vi "listenUDP.vi"(8 "error in (no error)":errorcluster, 11 "UDP Network Connection in":refnum<k16>) -> (0 "error out":errorcluster, 2 "data out":string, 3 "UDP Network Connection out":refnum<k16>)   [LabVIEW 2017, in "communicateMLC.lvlib"]
doc: "This VI listens for UDP data from the PC. The listening port is 60006."
uses:
  communicateMLC.lvlib
  TypeDefs/UDPListenFGV.ctl
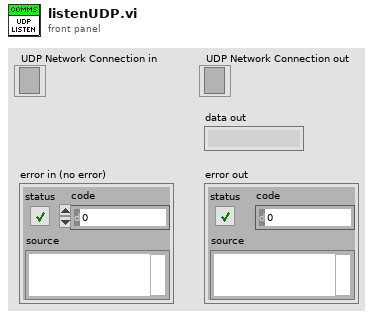
[diagram p1: front panel]
types:
  T1 = typedef "communicateMLC.lvlib/UDPListenFGV.ctl" = enum16{"Write", "Read"}
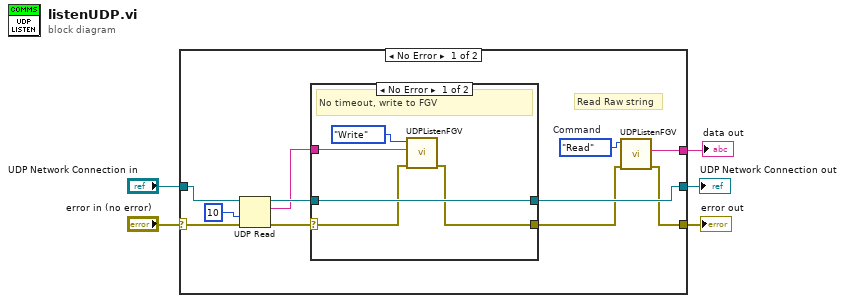
[diagram p0: block diagram]
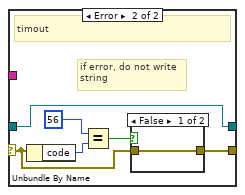
[diagram p2: hidden frame]
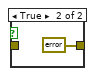
[diagram p3: hidden frame]
diagram:
  n1 = case shown="No Error" "error in (no error)" {
    selector: "error in (no error)" -> [w11 w31]
    tunnel: [w16 w30] -> w5
    tunnel: [w6 w31] -> w4
    tunnel: "UDP Network Connection in" -> [w15 w30]
    tunnel: [w8 _] -> w1
    frame No Error {
      w9 = UDPListenFGV."Read"  # Command
      # "Read Raw string"
      n2 = UDP Read(connection ID=w15, timeout ms (25000)=10, 8:w11) -> (data out=w10:string, error out=w13:errorcluster, 3:w14:refnum<k16>)  [unwired: 1 in, 2 out]
      n3 = case shown="No Error" w13 {
        selector: w13 -> [w20 w23]
        tunnel: w14 -> [w21 w22]
        tunnel: w10 -> [w18 _]
        tunnel: [w19 w24] -> w7
        tunnel: [w21 w22] -> w16
        frame No Error {
          # "No timeout, write to FGV"
          n4 = call "UDPListenFGV.vi"("error in (no error)"=w20, "Write Data"=w18, "Command"=UDPListenFGV."Write") -> ("error out"=w19:errorcluster)  [unwired: 7 in, 1 out]
        }
        frame Error {
          # "if error, do not write\nstring"
          # "timout"
          n5 = Unbundle By Name(w23) -> ("code"=w27:i32)
          n6 = Equal?(x=56, y=w27) -> (x = y?=w25:bool)
          n7 = case shown="False" w25 {
            tunnel: [w28 errorcluster {"status"=FALSE, "code"=0, "source"=""} ("error constant")] -> w24
            tunnel: w23 -> [w28 _]
            frame False {
            }
            frame True {
            }
          }
        }
      }
      n8 = call "UDPListenFGV.vi"("error in (no error)"=w7, "Command"=w9) -> ("error out"=w6:errorcluster, "Read Data"=w8:string)  [unwired: 8 in]
    }
    frame Error {
    }
  }
  "UDP Network Connection out" <- w5
  "error out" <- w4
  "data out" <- w1
